vi "HEWH Init_RLT_Equip.vi"(7 "Semiphore":T2, 8 "Error In":errorcluster, 9 "GEA?":bool, 10 "Agilent Channel Input":string, 11 "RLT Equipment":T1={"COM A"="COM3", "MW100"="MW100", "AG34970"="A-34972A", "COM B"="COM4", "COM C"="COM5", "COM D"="COM6"}) -> (0 "Error Out":errorcluster, 1 "Computer Name":string, 2 "LAN IP Address":string, 3 "RLT Equipment Out":T1={"COM A"="COM3", "MW100"="MW100", "AG34970"="A-34972A", "COM B"="COM4", "COM C"="COM5", "COM D"="COM6"}, 5 "InitOK":bool)   [LabVIEW 2012]
uses:
  <vilib>/Instr/_visa.llb/VISA Configure Serial Port (Instr).vi
panel:
  out "error cluster":T3
  # "GEA=19200 serial,\nMADEA = 9600 baud"
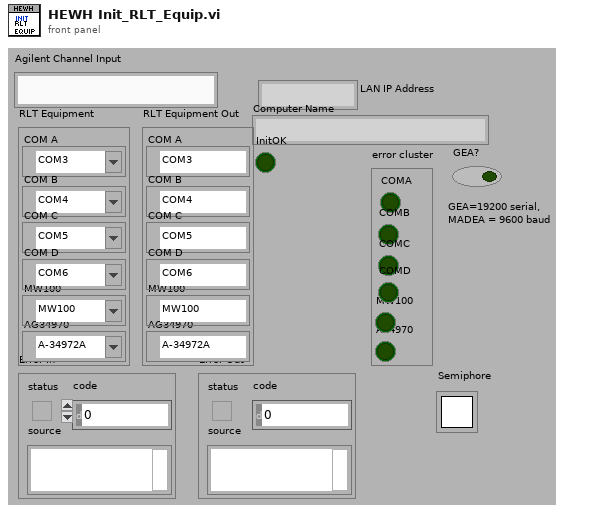
[diagram p1: front panel]
types:
  T1 = cluster{"COM A":refnum<visa-resource-name>, "MW100":refnum<visa-resource-name>, "AG34970":refnum<visa-resource-name>, "COM B":refnum<visa-resource-name>, "COM C":refnum<visa-resource-name>, "COM D":refnum<visa-resource-name>}
  T2 = typedef "Semaphore RefNum" = refnum<k1>
  T3 = cluster{"MW100":bool, "A34970":bool, "COMA":bool, "COMB":bool, "COMC":bool, "COMD":bool}
  T4 = enum16{"Computation Start", "Computation stop", "Reset Computation", "Clear Computation"}[]
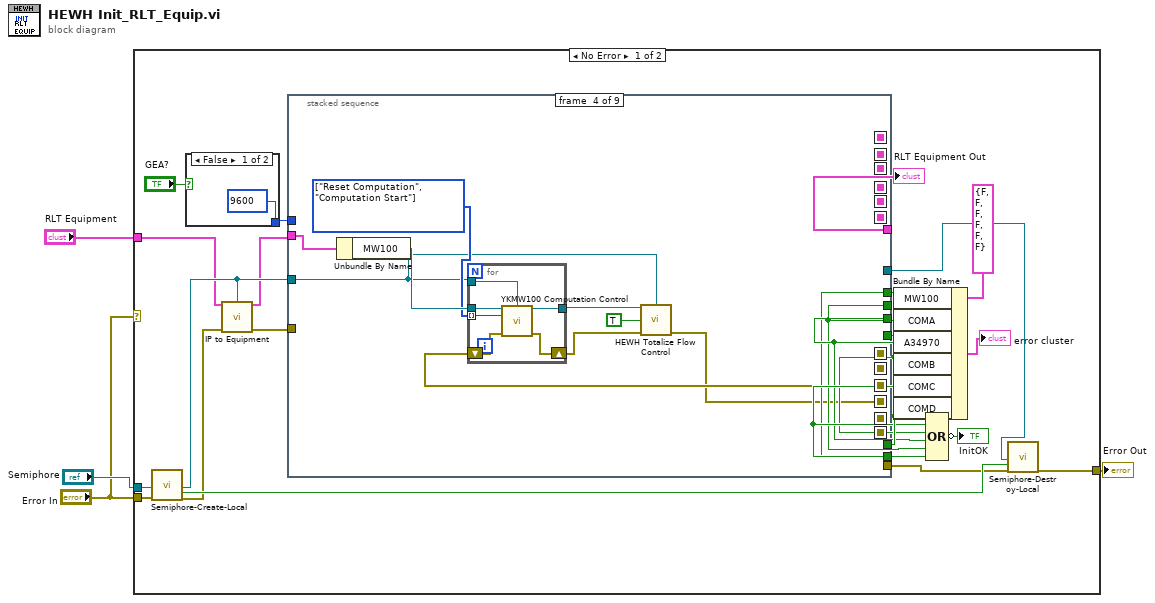
[diagram p0: block diagram]
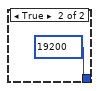
[diagram p2: hidden frame]
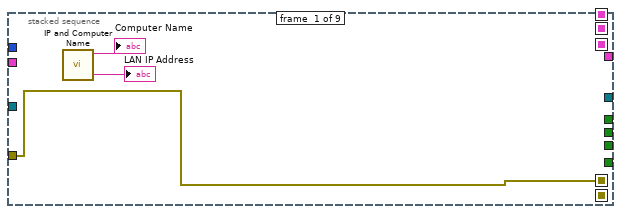
[diagram p3: hidden frame]
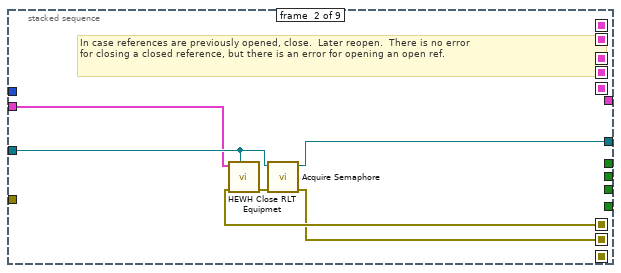
[diagram p4: hidden frame]
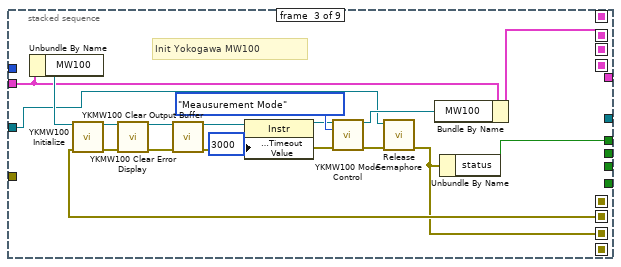
[diagram p5: hidden frame]
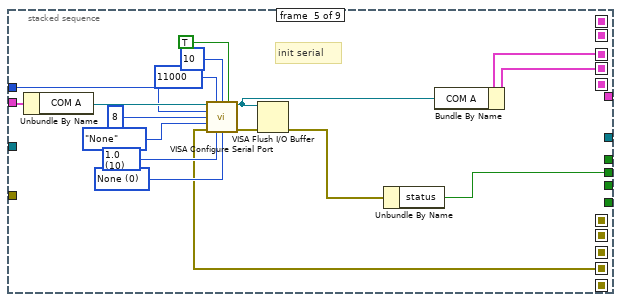
[diagram p6: hidden frame]
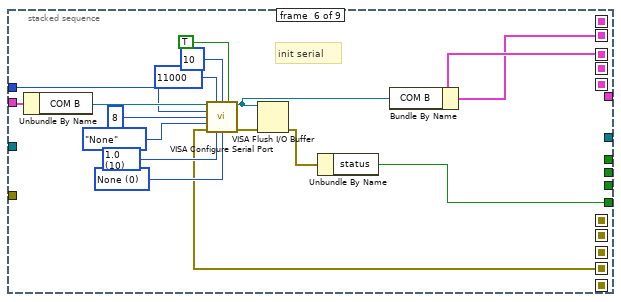
[diagram p7: hidden frame]
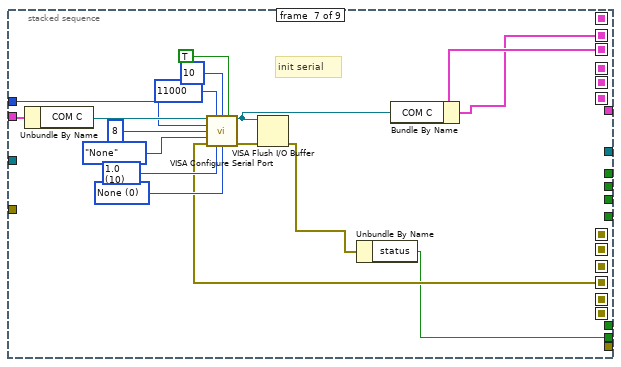
[diagram p8: hidden frame]
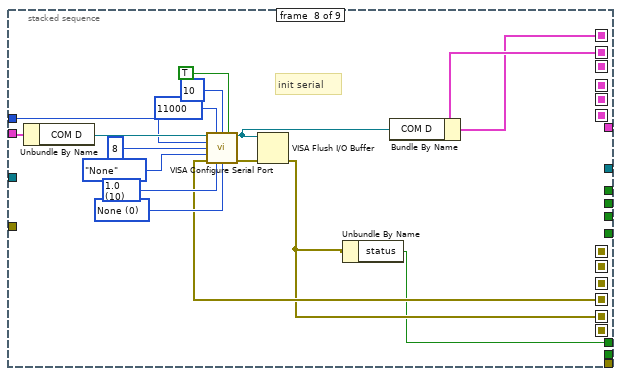
[diagram p9: hidden frame]
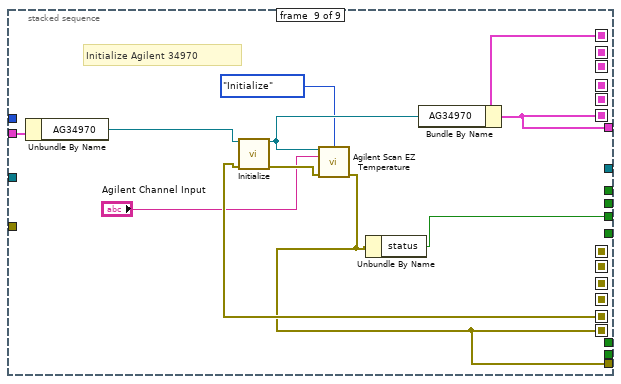
[diagram p10: hidden frame]
diagram:
  n1 = case shown="No Error" "Error In" {
    tunnel: "RLT Equipment" -> [w6 _]
    tunnel: "Semiphore" -> [w26 _]
    tunnel: "Error In" -> [w24 w152]
    tunnel: [w23 w152] -> w3
    frame No Error {
      n2 = call "Semiphore-Create-Local.vi"("Semiphore"=w26, "error in (no error)"=w24) -> ("semaphore"=w7:T2, "Local?"=w25:bool, "error out"=w8:errorcluster)  [unwired: 15 in]
      n3 = case shown="False" "GEA?" {
        tunnel: [u32 9600 ("baud rate (9600)") u32 19200 ("baud rate (9600)")] -> w11
        frame False {
        }
        frame True {
        }
      }
      n4 = call "IP to Equipment.vi"("RLT Equipment In"=w6, "MW100 Semiphore"=w7, "Error In"=w8) -> ("RLT Equip Out"=w5:T1, "Error Out"=w9:errorcluster)  [unwired: 10 in, 1 out]
      n5 = stacked-sequence {
        seq-local: [_ _ w39 _ _ _ _ _ _] -> [_ _ _ w66 _ _ _ _ _]
        seq-local: [_ _ _ _ _ _ _ w128 _] -> [_ _ _ _ _ _ _ _ w149]
        seq-local: [_ _ w56 _ _ _ _ _ _] -> [_ _ _ _ w83 w100 _ _ _]
        seq-local: [_ _ _ _ w82 _ _ _ _] -> [_ _ _ _ _ _ _ _ _]
        seq-local: [_ _ _ _ _ _ _ _ w141] -> [_ _ _ _ _ _ _ _ _]
        seq-local: [_ _ _ _ _ _ _ _ w143] -> [_ _ _ _ _ _ _ _ _]
        seq-local: [w30 _ _ _ _ _ _ _ _] -> [_ w36 _ _ _ _ _ _ _]
        seq-local: [_ w35 _ _ _ _ _ _ _] -> [_ _ w43 _ _ _ _ _ _]
        seq-local: [_ _ _ w60 _ _ _ _ _] -> [_ _ _ _ w74 w94 w112 w129 _]
        seq-local: [_ _ _ _ _ w91 _ _ _] -> [_ _ _ _ _ _ w109 _ _]
        seq-local: [_ _ _ _ _ _ w108 _ _] -> [_ _ _ _ _ _ _ w126 _]
        seq-local: [_ _ _ _ _ _ _ w125 _] -> [_ _ _ _ _ _ _ _ w142]
        tunnel: w9 -> [w30 _ _ _ _ _ _ _ _]
        tunnel: w5 -> [_ w34 w55 w65 w81 w99 w117 w134 w151]
        tunnel: [_ _ _ _ _ _ _ _ w143] -> w21
        tunnel: [_ _ w54 _ _ _ _ _ _] -> w13
        tunnel: [_ _ _ _ w79 _ _ _ _] -> w14
        tunnel: [_ _ _ _ _ _ _ _ w148] -> w15
        tunnel: w7 -> [_ w37 w40 w58 _ _ _ _ _]
        tunnel: [_ w33 _ _ _ _ _ _ _] -> w22
        tunnel: [_ _ _ _ _ w92 _ _ _] -> w16
        tunnel: [_ _ _ _ _ _ w110 _ _] -> w17
        tunnel: [_ _ _ _ _ _ _ w127 _] -> w18
        tunnel: [_ _ _ _ _ _ _ _ w141] -> w19
        tunnel: w11 -> [_ _ _ _ w73 w90 w107 w124 _]
        frame #0 {
          n6 = call "IP and Computer Name.vi"() -> ("IP Address"=→"LAN IP Address":string, "Computer Name"=→"Computer Name":string)  [unwired: 10 in]
        }
        frame #1 {
          # "In case references are previously opened, close.  Later reopen.  There is no error\nfor closing a closed reference, but there is an error for opening an open ref."
          n7 = call "HEWH Close RLT Equipmet.vi"("Semiphore"=w37, "Error In"=w36, "RLT Equipment"=w34) -> ("Error Out"=w38:errorcluster)  [unwired: 8 in]
          n8 = call <vilib>:"Acquire Semaphore.vi"("error in (no error)"=w38, "semaphore"=w37) -> ("error out"=w35:errorcluster, "semaphore out"=w33:T2)  [unwired: 3 in, 1 out]
        }
        frame #2 {
          # "Init Yokogawa MW100"
          n9 = Unbundle By Name(w55) -> ("MW100"=w57:refnum<visa-resource-name>)
          n10 = call "YKMW100 Initialize.vi"("VISA session (TCPIP::)"=w57, "error in (no error)"=w43) -> ("dup VISA session"=w44:refnum<visa-resource-name>, "error out"=w47:errorcluster)  [unwired: 12 in]
          n11 = call "YKMW100 Clear Error Display.vi"("VISA session"=w44, "error in (no error)"=w47) -> ("dup VISA session"=w45:refnum<visa-resource-name>, "error out"=w46:errorcluster)  [unwired: 10 in, 2 out]
          n12 = call "YKMW100 Clear Output Buffer.vi"("VISA session"=w45, "error in (no error)"=w46) -> ("dup VISA session"=w48:refnum<visa-resource-name>, "error out"=w49:errorcluster)  [unwired: 12 in]
          n13 = property class="Instr"(reference=w48, error in=w49, "General Settings:Timeout Value"=u32 3000) -> (reference out=w50:refnum<visa-resource-name>, error out=w51:errorcluster)
          n14 = call "YKMW100 Mode Control.vi"("VISA session"=w50, "Model"=enum16{"Meausurement Mode", "Setting Mode"}."Meausurement Mode", "error in (no error)"=w51) -> ("dup VISA session"=w42:refnum<visa-resource-name>, "error out"=w41:errorcluster)  [unwired: 11 in]
          n15 = call <vilib>:"Release Semaphore.vi"("error in (no error)"=w41, "semaphore"=w40) -> ("error out"=w39:errorcluster)  [unwired: 4 in, 1 out]
          n16 = Bundle By Name(cluster=w55, "MW100"=w42) -> (w56:T1)
          n17 = Unbundle By Name(w39) -> ("status"=w54:bool)
        }
        frame #3 {
          w63 = T4 [enum."Reset Computation", enum."Computation Start"] items=["Computation Start", "Computation stop", "Reset Computation", "Clear Computation"]
          n18 = Unbundle By Name(w65) -> ("MW100"=w64:refnum<visa-resource-name>)
          n19 = for {
            tunnel: w58 -> [w70]
            tunnel: w64 -> [w69]
            tunnel: w63 -> [w68] mode=indexing
            shift-right: [w71] -> w61
            shift-left: w66 -> [w72]
            tunnel: [w67] -> w59
            n20 = call "YKMW100 Computation Control.vi"("VISA session"=w69, "Semiphore"=w70, "Mode"=w68, "error in (no error)"=w72) -> ("dup VISA session"=w67:refnum<visa-resource-name>, "error out"=w71:errorcluster)  [unwired: 10 in]
          }
          n21 = call "HEWH Totalize Flow Control.vi"("VISA session"=w59, "Semiphore"=w58, "Totalize Flow"=TRUE, "error in (no error)"=w61) -> ("error out"=w60:errorcluster)  [unwired: 10 in, 1 out]
        }
        frame #4 {
          w86 = u16 0 items=["None", "XON/XOFF", "RTS/CTS", "XON/XOFF & RTS/CTS", "DTR/DSR", "XON/XOFF & DTR/DSR"] ("flow control (0:none)")
          w87 = u16 10 items=["1.0"=10, "1.5"=15, "2.0"=20] ("stop bits (10: 1 bit)")
          # "init serial"
          n22 = Unbundle By Name(w81) -> ("COM A"=w80:refnum<visa-resource-name>)
          n23 = call-poly "VISA Configure Serial Port"("VISA resource name"=w80, "timeout (10sec)"=u32 11000, "termination char\n(0xA = '\\n' = LF)"=u8 10 ("termination char\n(0xA = '\\n' = LF)"), "Enable Termination\nChar (T)"=TRUE ("Enable Termination\nChar (T)"), "baud rate (9600)"=w73, "data bits (8)"=u16 8, "parity (0:none)"=enum16{"None", "Odd", "Even", "Mark", "Space"}."None", "error in (no error)"=w74, "stop bits (10: 1 bit)"=w87, "flow control (0:none)"=w86) -> ("VISA resource name out"=w75:refnum<visa-resource-name>, "error out"=w77:errorcluster)  [unwired: 4 in]
          n24 = VISA Flush I/O Buffer(VISA resource name=w75, error in (no error)=w77) -> (error out=w76:errorcluster)  [unwired: 1 in, 1 out]
          n25 = Unbundle By Name(w76) -> ("status"=w79:bool)
          n26 = Bundle By Name(cluster=w83, "COM A"=w75) -> (w82:T1)
        }
        frame #5 {
          w103 = u16 0 items=["None", "XON/XOFF", "RTS/CTS", "XON/XOFF & RTS/CTS", "DTR/DSR", "XON/XOFF & DTR/DSR"] ("flow control (0:none)")
          w104 = u16 10 items=["1.0"=10, "1.5"=15, "2.0"=20] ("stop bits (10: 1 bit)")
          # "init serial"
          n27 = Unbundle By Name(w99) -> ("COM B"=w98:refnum<visa-resource-name>)
          n28 = call-poly "VISA Configure Serial Port"("VISA resource name"=w98, "timeout (10sec)"=u32 11000, "termination char\n(0xA = '\\n' = LF)"=u8 10 ("termination char\n(0xA = '\\n' = LF)"), "Enable Termination\nChar (T)"=TRUE ("Enable Termination\nChar (T)"), "baud rate (9600)"=w90, "data bits (8)"=u16 8, "parity (0:none)"=enum16{"None", "Odd", "Even", "Mark", "Space"}."None", "error in (no error)"=w94, "stop bits (10: 1 bit)"=w104, "flow control (0:none)"=w103) -> ("VISA resource name out"=w95:refnum<visa-resource-name>, "error out"=w96:errorcluster)  [unwired: 4 in]
          n29 = VISA Flush I/O Buffer(VISA resource name=w95, error in (no error)=w96) -> (error out=w93:errorcluster)  [unwired: 1 in, 1 out]
          n30 = Unbundle By Name(w93) -> ("status"=w92:bool)
          n31 = Bundle By Name(cluster=w100, "COM B"=w95) -> (w91:T1)
        }
        frame #6 {
          w120 = u16 0 items=["None", "XON/XOFF", "RTS/CTS", "XON/XOFF & RTS/CTS", "DTR/DSR", "XON/XOFF & DTR/DSR"] ("flow control (0:none)")
          w121 = u16 10 items=["1.0"=10, "1.5"=15, "2.0"=20] ("stop bits (10: 1 bit)")
          # "init serial"
          n32 = Unbundle By Name(w117) -> ("COM C"=w116:refnum<visa-resource-name>)
          n33 = call-poly "VISA Configure Serial Port"("VISA resource name"=w116, "timeout (10sec)"=u32 11000, "termination char\n(0xA = '\\n' = LF)"=u8 10 ("termination char\n(0xA = '\\n' = LF)"), "Enable Termination\nChar (T)"=TRUE ("Enable Termination\nChar (T)"), "baud rate (9600)"=w107, "data bits (8)"=u16 8, "parity (0:none)"=enum16{"None", "Odd", "Even", "Mark", "Space"}."None", "error in (no error)"=w112, "stop bits (10: 1 bit)"=w121, "flow control (0:none)"=w120) -> ("VISA resource name out"=w113:refnum<visa-resource-name>, "error out"=w114:errorcluster)  [unwired: 4 in]
          n34 = VISA Flush I/O Buffer(VISA resource name=w113, error in (no error)=w114) -> (error out=w111:errorcluster)  [unwired: 1 in, 1 out]
          n35 = Unbundle By Name(w111) -> ("status"=w110:bool)
          n36 = Bundle By Name(cluster=w109, "COM C"=w113) -> (w108:T1)
        }
        frame #7 {
          w137 = u16 0 items=["None", "XON/XOFF", "RTS/CTS", "XON/XOFF & RTS/CTS", "DTR/DSR", "XON/XOFF & DTR/DSR"] ("flow control (0:none)")
          w138 = u16 10 items=["1.0"=10, "1.5"=15, "2.0"=20] ("stop bits (10: 1 bit)")
          # "init serial"
          n37 = Unbundle By Name(w134) -> ("COM D"=w133:refnum<visa-resource-name>)
          n38 = call-poly "VISA Configure Serial Port"("VISA resource name"=w133, "timeout (10sec)"=u32 11000, "termination char\n(0xA = '\\n' = LF)"=u8 10 ("termination char\n(0xA = '\\n' = LF)"), "Enable Termination\nChar (T)"=TRUE ("Enable Termination\nChar (T)"), "baud rate (9600)"=w124, "data bits (8)"=u16 8, "parity (0:none)"=enum16{"None", "Odd", "Even", "Mark", "Space"}."None", "error in (no error)"=w129, "stop bits (10: 1 bit)"=w138, "flow control (0:none)"=w137) -> ("VISA resource name out"=w130:refnum<visa-resource-name>, "error out"=w131:errorcluster)  [unwired: 4 in]
          n39 = VISA Flush I/O Buffer(VISA resource name=w130, error in (no error)=w131) -> (error out=w128:errorcluster)  [unwired: 1 in, 1 out]
          n40 = Unbundle By Name(w128) -> ("status"=w127:bool)
          n41 = Bundle By Name(cluster=w126, "COM D"=w130) -> (w125:T1)
        }
        frame #8 {
          # "Initialize Agilent 34970"
          n42 = Unbundle By Name(w151) -> ("AG34970"=w150:refnum<visa-resource-name>)
          n43 = call <instrlib>:"Initialize.vi"("VISA Resource Name"=w150, "error in (no error)"=w149) -> ("VISA Resource Name Out"=w146:refnum<visa-resource-name>, "error out"=w147:errorcluster)  [unwired: 12 in]
          n44 = call "Agilent Scan EZ Temperature.vi"("VISA Resource Name"=w146, "Control"=enum16{"Initialize", "Read", "Experiment"}."Initialize", "Channel Input"="Agilent Channel Input", "error in (no error)"=w147) -> ("error out"=w143:errorcluster)  [unwired: 8 in, 3 out]
          n45 = Unbundle By Name(w143) -> ("status"=w148:bool)
          n46 = Bundle By Name(cluster=w142, "AG34970"=w146) -> (w141:T1)
        }
      }
      "RLT Equipment Out" <- w19
      n47 = Bundle By Name(cluster=T3 {"MW100"=FALSE, "A34970"=FALSE, "COMA"=FALSE, "COMB"=FALSE, "COMC"=FALSE, "COMD"=FALSE} ("error cluster 2"), "MW100"=w13, "COMA"=w14, "A34970"=w15, "COMB"=w16, "COMC"=w17, "COMD"=w18) -> (→"error cluster":T3)
      n48 = Compound Arithmetic op=OR(w18, w17, w16, w15, w14, w13) -> (invert →"InitOK":bool)
      n49 = call "Semiphore-Destroy-Local.vi"("Semiphore"=w22, "Local?"=w25, "error in (no error)"=w21) -> ("error out"=w23:errorcluster)  [unwired: 16 in]
    }
    frame Error {
    }
  }
  "Error Out" <- w3
